vi "Rotating a Picture.vi"() -> ()   [LabVIEW 2023]
doc: "Demonstrates how to rotate an image displayed in a 2D Picture. This feature is important when you want to animate the state of an object, like the attitude of an airplane."
uses:
  <vilib>/picture/picture.llb/Draw True-Color Pixmap.vi
panel:
  in  "Scale":dbl(slide)=1.0 scale=0.1..10.0
  in  "Stop":bool
  in  "Rotation Angle (radians)":dbl(knob) scale=-3.14..3.14
  out "2D Picture":picture
  # "Overview: This VI demonstrates how to rotate and scale an image displayed in a 2D Picture.\nInstructions: \n1. Run the VI. \n2. Change the Scale and Rotation Angle of the image and observe the change in the displayed image.\n3. Click Stop to stop the VI."
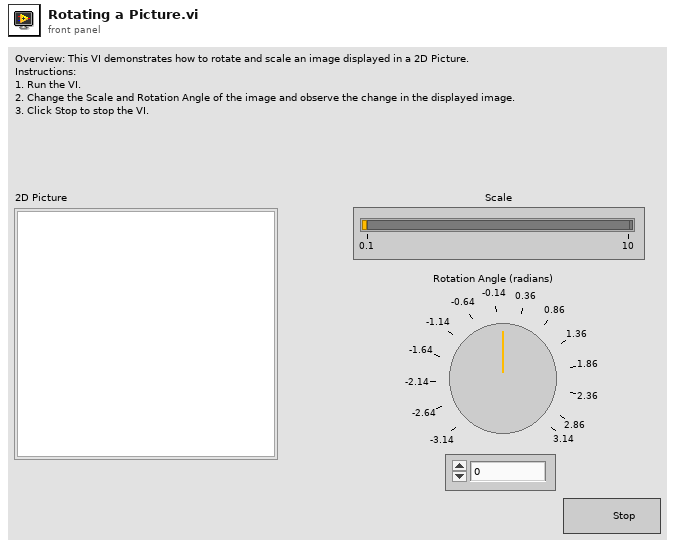
[diagram p1: front panel]
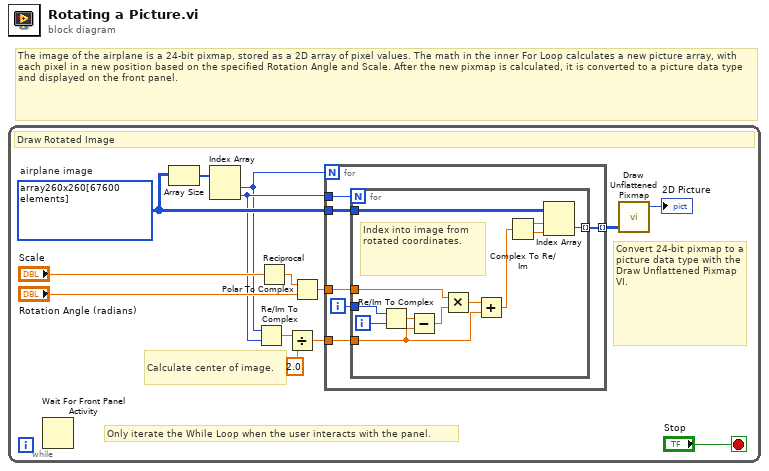
[diagram p0: block diagram]
diagram:
  # "The image of the airplane is a 24-bit pixmap, stored as a 2D array of pixel values. The math in the inner For Loop calculates a new picture array, with each pixel in a new position based on the specified Rotation Angle and Scale. After the new pixmap is calculated, it is converted to a picture data type and displayed on the front panel."
  n1 = while {
    stop <- "Stop" stop-if-true
    w13 = u32[][] array260x260[67600 elements]  # airplane image
    # "Calculate center of image."
    # "Only iterate the While Loop when the user interacts with the panel."
    # "Convert 24-bit pixmap to a picture data type with the Draw Unflattened Pixmap VI."
    # "Draw Rotated Image"
    n2 = Wait For Front Panel Activity() -> ()  [unwired: 3 in, 1 out]
    n3 = Array Size(array=w13) -> (size(s)=w5:i32[])
    n4 = Index Array(array=w5) -> (element #1=w3:i32, element #2=w4:i32)  [unwired: 2 in]
    n5 = Re/Im To Complex(1:w4, 2:w3) -> (0:w6:cdb)
    n6 = Reciprocal(x="Scale") -> (1/x=w8:dbl)
    n7 = Divide(x=w6, y=2.0) -> (x/y=w2:cdb)
    n8 = Polar To Complex(1:"Rotation Angle (radians)", 2:w8) -> (0:w7:cdb)
    n9 = for {
      N: w3 -> [_]
      tunnel: w4 -> [w19]
      tunnel: w13 -> [w18]
      tunnel: [w17] -> w14 mode=indexing
      tunnel: w7 -> [w16]
      tunnel: w2 -> [w15]
      i -> [w20]
      n10 = for {
        N: w19 -> [_]
        tunnel: w20 -> [w29]
        tunnel: w18 -> [w32]
        tunnel: [w31] -> w17 mode=indexing
        tunnel: w16 -> [w26]
        tunnel: w15 -> [w21]
        i -> [w30]
        # "Index into image from rotated coordinates."
        n11 = Re/Im To Complex(1:w30, 2:w29) -> (0:w28:cdb)
        n12 = Subtract(x=w28, y=w21) -> (x-y=w27:cdb)
        n13 = Multiply(x=w26, y=w27) -> (x*y=w25:cdb)
        n14 = Add(x=w25, y=w21) -> (x+y=w24:cdb)
        n15 = Complex To Re/Im(x + iy=w24) -> (x=w23:dbl, y=w22:dbl)
        n16 = Index Array(array=w32, index (row)=w23, index (col)=w22) -> (element=w31:u32)
      }
    }
    n17 = call-poly <vilib>:"Draw Unflattened Pixmap.vi"("data (RGB format)"=w14) -> ("new picture"=→"2D Picture":picture)  [unwired: 8 in]
  }
